vi "联动声光报警(子VI).vi"(11 "布尔":bool) -> ()   [LabVIEW 2016, in "环境动力监测库.lvlib"]
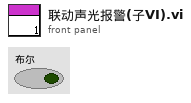
[diagram p1: front panel]
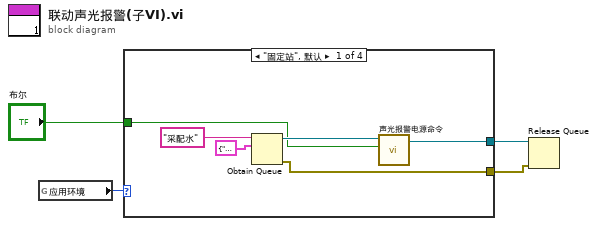
[diagram p0: block diagram]
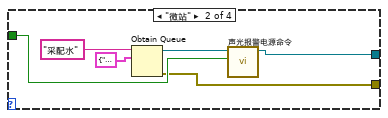
[diagram p2: hidden frame]
diagram:
  n1 = global read "外部交互全局变量.vi" "应用环境"() -> (w4:enum16{"固定站", "微站", "浮标", "浮船"})
  n2 = case shown="\"固定站\", 默认" w4 {
    tunnel: "布尔" -> [w7 w13 _ _]
    tunnel: [w6 w12 _ _] -> w2
    tunnel: [w5 w11 _ _] -> w1
    frame "固定站", Default {
      n3 = Obtain Queue(name (unnamed)="采配水" ("名称（未命名）"), element data type=cluster{"命令":string, "数据":variant} {"命令"="", "数据"=variant}) -> (queue out=w8:refnum<queue>, error out=w5:errorcluster)  [unwired: 3 in, 1 out]
      n4 = call "声光报警电源命令.vi"("通电/断电"=w7, "队列"=w8) -> ("队列输出"=w6:refnum<queue>)  [unwired: 9 in]
    }
    frame "微站" {
      n5 = Obtain Queue(name (unnamed)="采配水" ("名称（未命名）"), element data type=cluster{"命令":string, "数据":variant} {"命令"="", "数据"=variant}) -> (queue out=w14:refnum<queue>, error out=w11:errorcluster)  [unwired: 3 in, 1 out]
      n6 = call "声光报警电源命令.vi"("通电/断电"=w13, "队列"=w14) -> ("队列输出"=w12:refnum<queue>)  [unwired: 9 in]
    }
    frame "浮标" {
    }
    frame "浮船" {
    }
  }
  n7 = Release Queue(queue=w2, error in (no error)=w1) -> ()  [unwired: 1 in, 3 out]
